vi "TcA05-001_ImplementingInterfaces.vi"(1 "Input buffer":T3="1", 3 "Invocation info":T2, 5 "error in (no error)":errorcluster, 6 "Add log to result?":bool) -> (16 "Test Data":T1 {"Numeric Measurement" format="%.2f"}, 19 "error out":errorcluster)   [LabVIEW 2020]
doc: "Test case template."
uses:
  Shared/Support_InputBuffer.ctl
  Shared/Support_InvocationInfo.ctl
  Shared/Support_TestData.ctl
  TestClasses/G#BaseClass2_class/G#BaseClass2.lvclass
  C:/Program Files (x86)/National Instruments/LabVIEW 2020/vi.lib/addons/_AddQ/G#Object/G#Object.lvclass
  TestClasses/G#SubClass2_class/G#SubClass2.lvclass
  TestClasses/G#BaseClass1_class/G#BaseClass1.lvclass
  TestClasses/G#BaseClass2_class/interfaces/G#BaseClass2_IG#BaseInterface/G#BaseClass2_IG#BaseInterface.lvclass
  C:/Projects/GsharpGIT/Verification/TestCases/TestClasses/IG#BaseInterface_interface/IG#BaseInterface.lvclass
  TestClasses/G#BaseClass1_class/interfaces/G#BaseClass1_IG#BaseInterface/G#BaseClass1_IG#BaseInterface.lvclass
  TestClasses/IG#BaseInterface_interface/IG#BaseInterface.lvclass
  <vilib>/addons/_AddQ/G#Object/G#Object.lvclass
panel:
  in  "Test name":string="TcA05-001 Implementing Interfaces"
  out "Test result":bool
  out "Result":string
  # "Verifying that the interface implementation works."
  # "Sub test case"
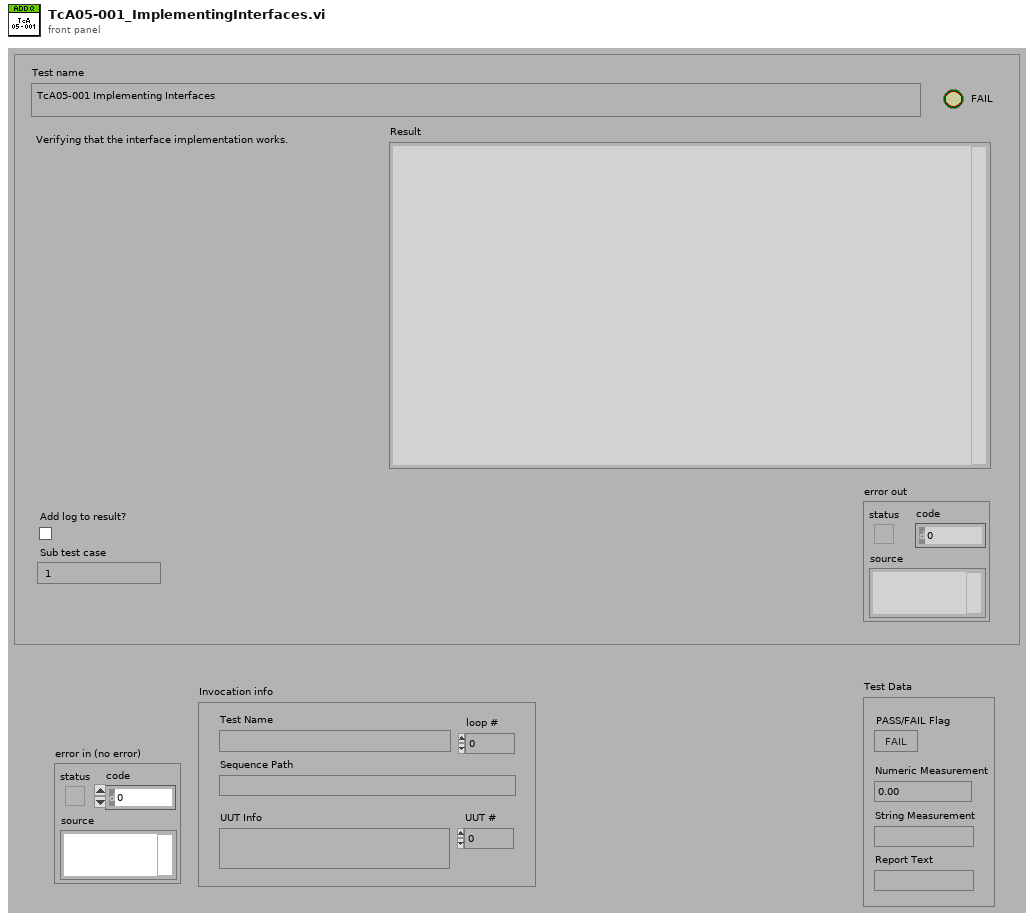
[diagram p1: front panel]
types:
  T1 = typedef "Support_TestData.ctl" = cluster{"PASS/FAIL Flag":bool, "Numeric Measurement":dbl, "String Measurement":string, "Report Text":string}
  T2 = typedef "Support_InvocationInfo.ctl" = cluster{"UUT #":i32, "loop #":i32, "UUT Info":string, "Test Name":string, "Sequence Path":path}
  T3 = typedef "Support_InputBuffer.ctl" = string
  T4 = typedef "Support_ResultType.ctl" = cluster{"Pass":bool, "Comment":string, "MeasurementValue":dbl}
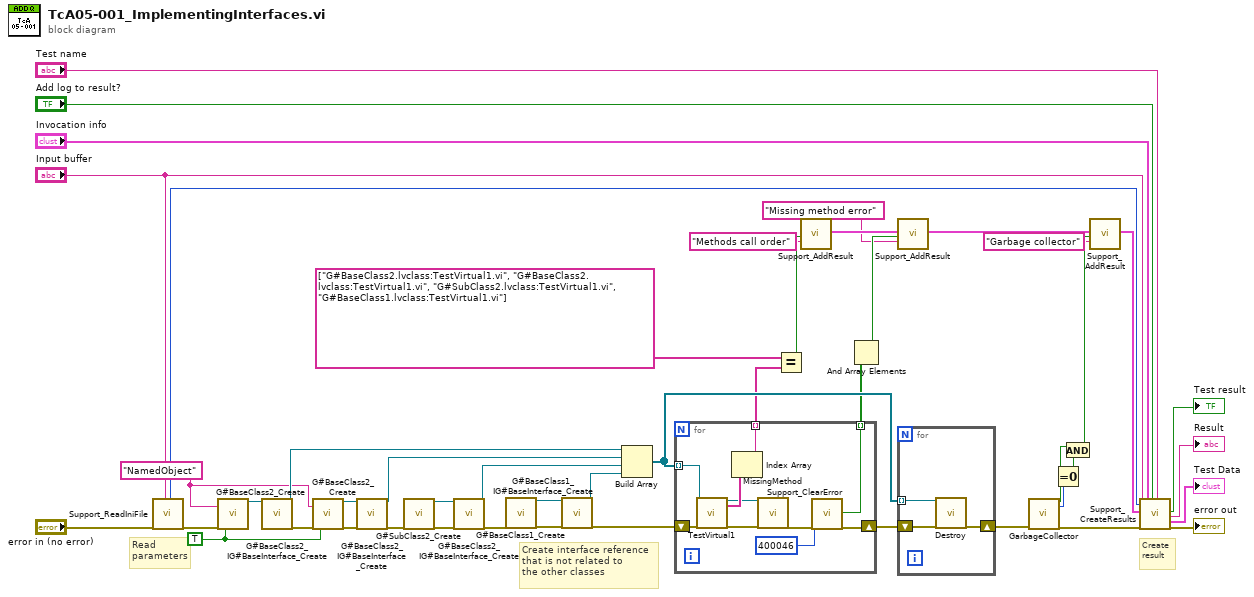
[diagram p0: block diagram]
diagram:
  w1 = "NamedObject" ("object name")
  w4 = TRUE ("user counter")
  # "Create interface reference\nthat is not related to\nthe other classes"
  # "Create\nresult"
  # "Read\nparameters"
  n1 = call "Support_ReadIniFile.vi"("error in (no error)"="error in (no error)", "Sub test case"="Input buffer") -> ("Timer start"=w37:u32, "error out"=w5:errorcluster)  [unwired: 10 in, 6 out]
  n2 = call "G#BaseClass2_Create.vi"("object name"=w1, "error in (no error)"=w5, "user counter"=w4) -> ("reference out"=w7:refnum<class "G#BaseClass2.lvclass">)  [unwired: 15 in, 1 out]
  n3 = call "G#BaseClass2_IG#BaseInterface_Create.vi"("reference in"=w7) -> ("reference out"=w3:refnum<class "G#BaseClass2_IG#BaseInterface.lvclass">, "error out"=w6:errorcluster)  [unwired: 17 in]
  n4 = call "G#BaseClass2_Create.vi"("object name"=w1, "error in (no error)"=w6, "user counter"=w4) -> ("reference out"=w34:refnum<class "G#BaseClass2.lvclass">, "error out"=w35:errorcluster)  [unwired: 15 in]
  n5 = call "G#BaseClass2_IG#BaseInterface_Create.vi"("reference in"=w34, "error in (no error)"=w35) -> ("reference out"=w26:refnum<class "G#BaseClass2_IG#BaseInterface.lvclass">, "error out"=w32:errorcluster)  [unwired: 16 in]
  n6 = call "G#SubClass2_Create.vi"("error in (no error)"=w32) -> ("reference out"=w31:refnum<class "G#SubClass2.lvclass">, "error out"=w33:errorcluster)  [unwired: 17 in]
  n7 = call "G#BaseClass2_IG#BaseInterface_Create.vi"("reference in"=w31, "error in (no error)"=w33) -> ("reference out"=w25:refnum<class "G#BaseClass2_IG#BaseInterface.lvclass">, "error out"=w30:errorcluster)  [unwired: 16 in]
  n8 = call "G#BaseClass1_Create.vi"("error in (no error)"=w30) -> ("reference out"=w28:refnum<class "G#BaseClass1.lvclass">, "error out"=w29:errorcluster)  [unwired: 16 in, 1 out]
  n9 = call "G#BaseClass1_IG#BaseInterface_Create.vi"("reference in"=w28, "error in (no error)"=w29) -> ("reference out"=w24:refnum<class "G#BaseClass1_IG#BaseInterface.lvclass">, "error out"=w27:errorcluster)  [unwired: 16 in]
  n10 = Build Array(w3, w26, w25, w24) -> (w22:refnum<class "IG#BaseInterface.lvclass">[])
  n11 = for {
    tunnel: w22 -> [w55] mode=indexing
    shift-right: [w53] -> w23
    shift-left: w27 -> [w57]
    tunnel: [w49] -> w15 mode=indexing
    tunnel: [w48] -> w10 mode=indexing
    n12 = call-dynamic "TestVirtual1.vi"("reference in"=w55, "error in (no error)"=w57) -> ("reference out"=w51:refnum<class "IG#BaseInterface.lvclass">, "MethodName"=w52:string[], "error out"=w56:errorcluster)  [unwired: 15 in]
    n13 = Index Array(array=w52) -> (element=w49:string)  [unwired: 1 in]
    n14 = call-dynamic "MissingMethod.vi"("reference in"=w51, "error in (no error)"=w56) -> ("error out"=w54:errorcluster)  [unwired: 16 in, 1 out]
    n15 = call "Support_ClearError.vi"("code"=400046, "error in (no error)"=w54) -> ("Cleared?"=w48:bool, "error out"=w53:errorcluster)  [unwired: 16 in]
  }
  n16 = Equal?(x=string[] ["G#BaseClass2.lvclass:TestVirtual1.vi", "G#BaseClass2.lvclass:TestVirtual1.vi", "G#SubClass2.lvclass:TestVirtual1.vi", "G#BaseClass1.lvclass:TestVirtual1.vi"] ("Array"), y=w15) -> (x = y?=w14:bool)
  n17 = call "Support_AddResult.vi"("Pass"=w14, "Comment"="Methods call order") -> ("Results out"=w12:T4[])  [unwired: 17 in]
  n18 = And Array Elements(Boolean array=w10) -> (logical AND=w9:bool)
  n19 = call "Support_AddResult.vi"("Results in"=w12, "Pass"=w9, "Comment"="Missing method error") -> ("Results out"=w11:T4[])  [unwired: 16 in]
  n20 = for {
    tunnel: w22 -> [w59] mode=indexing
    shift-right: [w58] -> w21
    shift-left: w23 -> [w60]
    n21 = call-dynamic "Destroy.vi"("reference in"=w59, "error in (no error)"=w60) -> ("error out"=w58:errorcluster)  [unwired: 16 in, 1 out]
  }
  n22 = call <vilib>:"GarbageCollector.vi"("error in (no error)"=w21) -> ("OK"=w19:bool, "# of objects killed"=w20:i32, "error out"=w36:errorcluster)  [unwired: 16 in]
  n23 = Equal To 0?(x=w20) -> (x = 0?=w18:bool)
  n24 = And(x=w19, y=w18) -> (x .and. y?=w17:bool)
  n25 = call "Support_AddResult.vi"("Results in"=w11, "Pass"=w17, "Comment"="Garbage collector") -> ("Results out"=w40:T4[])  [unwired: 16 in]
  n26 = call "Support_CreateResults.vi"("Sub test case"="Input buffer", "Timer start"=w37, "Results"=w40, "error in (no error)"=w36, "Invocation info"="Invocation info", "Add log to result?"="Add log to result?", "Test name"="Test name") -> ("Pass/fail flag"=→"Test result":bool, "Result"=→"Result":string, "Test Data"=→"Test Data":T1, "error out"=→"error out":errorcluster)  [unwired: 9 in]
